vi "setShifts.vi"(8 "error in (no error)":errorcluster, 10 "shifts":refnum<class "Shift.lvclass">[](array[class]), 11 "Shift Schedule in":refnum<class "Shift Schedule.lvclass">) -> (0 "error out":errorcluster, 3 "Shift Schedule out":refnum<class "Shift Schedule.lvclass">)   [LabVIEW 2013, in "Shift Schedule.lvclass"]
uses:
  Shift Schedule.lvclass
  Shift.lvclass
  Shift Schedule.lvclass/Shift Schedule.ctl
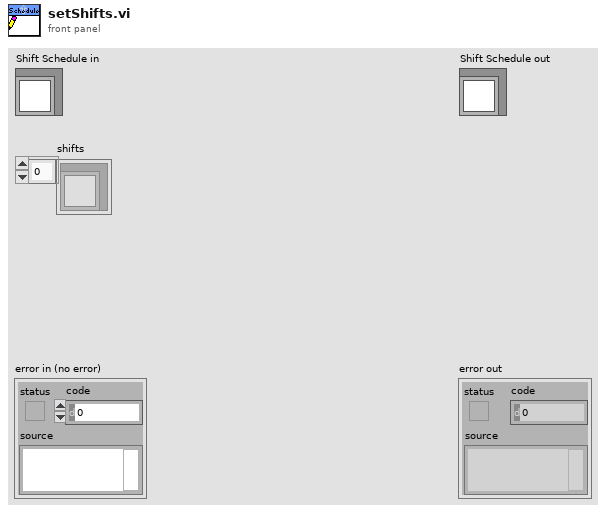
[diagram p1: front panel]
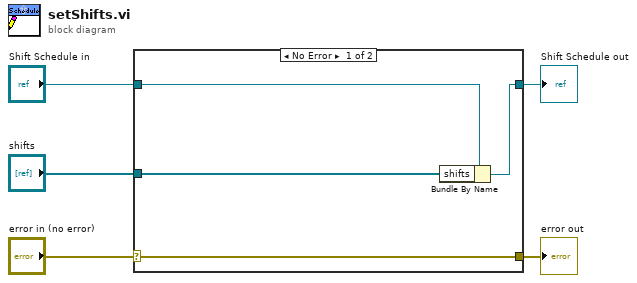
[diagram p0: block diagram]
diagram:
  n1 = case shown="No Error" "error in (no error)" {
    selector: "error in (no error)" -> [w9 w10]
    tunnel: [w9 w10] -> w4
    tunnel: [w7 w11] -> w2
    tunnel: "Shift Schedule in" -> [w8 w11]
    tunnel: "shifts" -> [w6 _]
    frame No Error {
      n2 = Bundle By Name(cluster=w8, "shifts"=w6) -> (w7:refnum<class "Shift Schedule.lvclass">)
    }
    frame Error {
    }
  }
  "error out" <- w4
  "Shift Schedule out" <- w2
